vi "Pump Status.vi"(8 "error in":errorcluster, 11 "Masterflex 75211 Settings":T1) -> (0 "error out":errorcluster, 1 "Connection Error":bool, 2 "Pump On?":enum16{"Off", "On", "Not Initialized"}(ring), 3 "Masterflex 75211 Settings":T1)   [LabVIEW 2018, in "Masterflex 75211.lvlib"]
uses:
  Masterflex 75211.lvlib
  Masterflex 75211 DAQ Setting.ctl
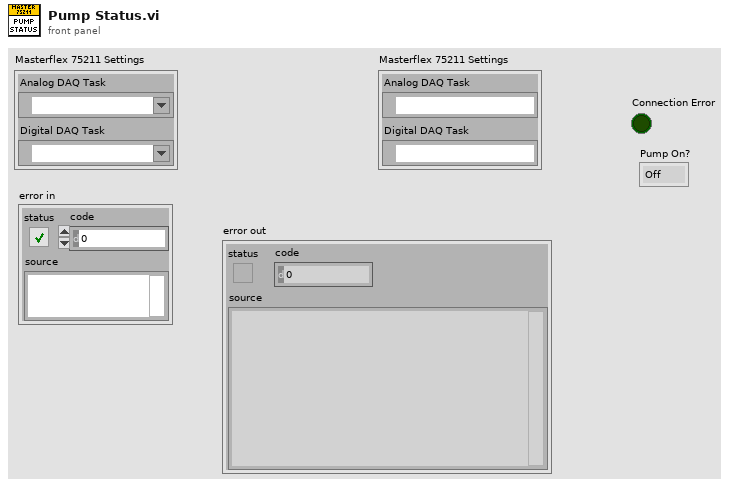
[diagram p1: front panel]
types:
  T1 = typedef "Masterflex 75211.lvlib/Masterflex 75211 DAQ Setting.ctl" = cluster{"Analog DAQ Task":refnum<k21>, "Digital DAQ Task":refnum<k21>}
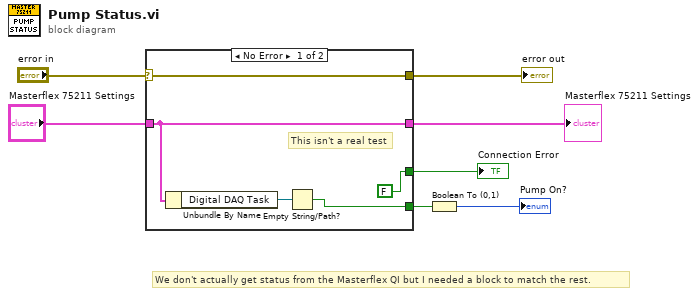
[diagram p0: block diagram]
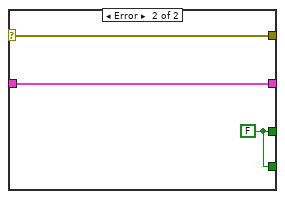
[diagram p2: hidden frame]
diagram:
  # "We don't actually get status from the Masterflex QI but I needed a block to match the rest."
  n1 = case shown="No Error" "error in" {
    selector: "error in" -> [w12 w14]
    tunnel: [w12 w14] -> w6
    tunnel: "Masterflex 75211 Settings" -> [w10 w15]
    tunnel: [w10 w15] -> w1
    tunnel: [FALSE w13] -> w5
    tunnel: [w8 w13] -> w3
    frame No Error {
      # "This isn't a real test"
      n2 = Unbundle By Name(w10) -> ("Digital DAQ Task"=w9:refnum<k21>)
      n3 = Empty String/Path?(string/path=w9) -> (empty?=w8:bool)
    }
    frame Error {
      w13 = FALSE
    }
  }
  "error out" <- w6
  "Connection Error" <- w5
  "Masterflex 75211 Settings" <- w1
  n4 = Boolean To (0,1)(Boolean=w3) -> (0, 1=→"Pump On?":i16)
